vi "UnregisterCEPMLocalFeed.vi"(8 "Error In":errorcluster) -> (0 "Error Out":errorcluster)   [LabVIEW 2019, in "CEPM.lvlib"]
uses:
  CEPM.lvlib
  <vilib>/National Instruments/NIPM API (Beta)/NIPM_API.lvlib
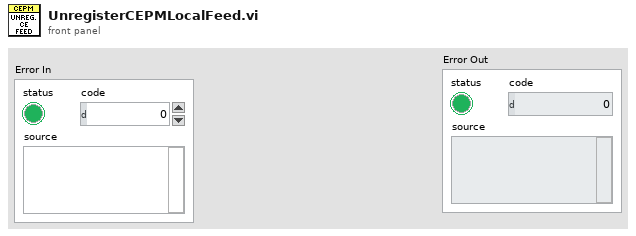
[diagram p1: front panel]
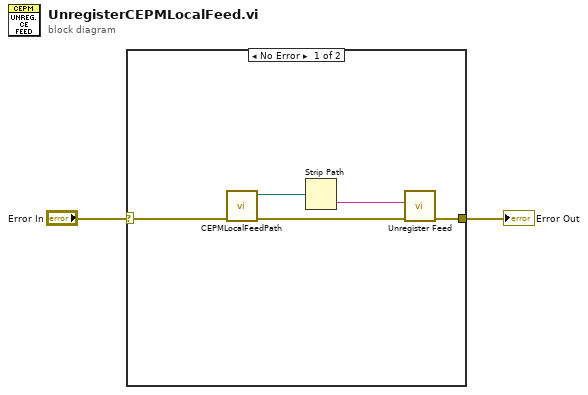
[diagram p0: block diagram]
diagram:
  n1 = case shown="No Error" "Error In" {
    selector: "Error In" -> [w6 w8]
    tunnel: [w7 w8] -> w1
    frame No Error {
      n2 = call "CEPMLocalFeedPath.vi"("Error In"=w6) -> ("Error Out"=w5:errorcluster, "CEPM Local Feed Path"=w4:path)  [unwired: 9 in]
      n3 = Strip Path(path=w4) -> (name=w3:string)  [unwired: 1 out]
      n4 = call <vilib>:"Unregister Feed.vi"("error in"=w5, "feed name"=w3) -> ("error out"=w7:errorcluster)  [unwired: 8 in, 1 out]
    }
    frame Error {
    }
  }
  "Error Out" <- w1
